vi "Ex_Inst_Read LabVIEW Measurement File.vi"(8 "error in (no error)":errorcluster, 9 "Filename":path, 10 "Enable":bool=TRUE, 11 "Reset":bool) -> (0 "error out":errorcluster, 2 "Filename Out":path, 3 "Signals":dynamicdata(graph), 4 "EOF?":bool, 5 "Comment":string, 7 "Description":string)   [LabVIEW 2017]
doc: "Reads data from a text-based measurement file (.lvm) or binary measurement file (.tdm or .tdms)."
uses:
  <vilib>/express/express shared/ExFile.llb/ex_FileFormats.ctl
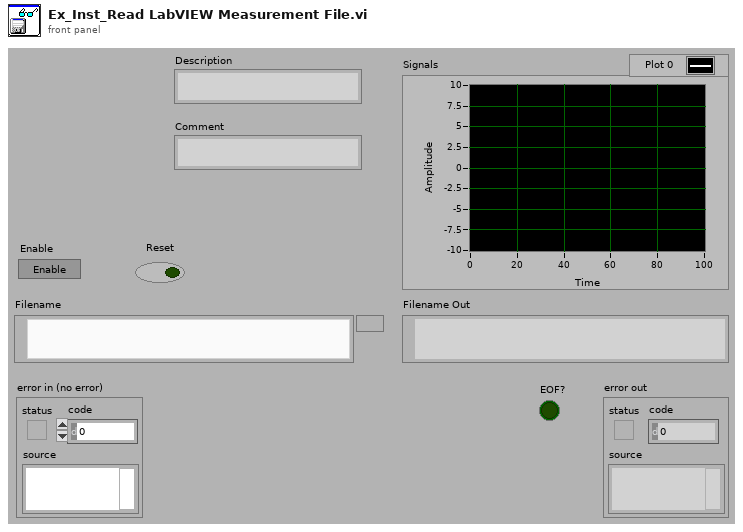
[diagram p1: front panel]
types:
  T1 = typedef "ex_FileFormats.ctl" = enum32{"lvm", "tdm", "tdms", "xlsx"}
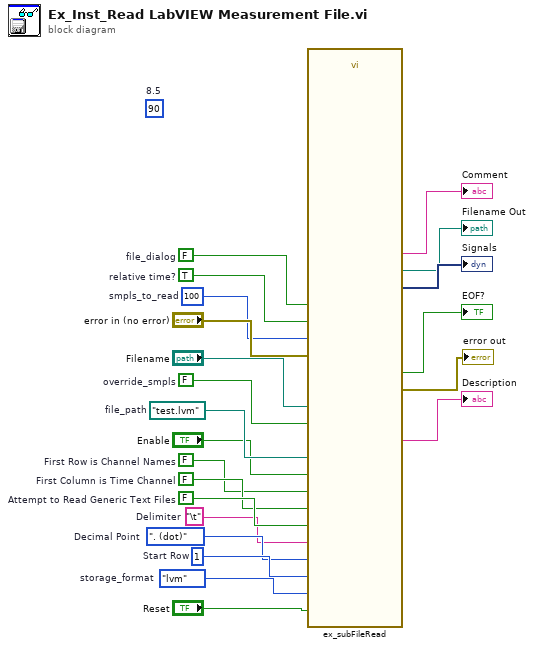
[diagram p0: block diagram]
diagram:
  (unwired) 90  # 8.5
  w4 = "\t"  # Delimiter
  w2 = ex_FileFormats."lvm"  # storage_format
  w5 = enum32{". (dot)", ", (comma)"}.". (dot)"  # Decimal Point
  w9 = 1  # Start Row
  w8 = FALSE  # Attempt to Read Generic Text Files
  w7 = FALSE  # First Column is Time Channel
  w6 = FALSE  # First Row is Channel Names
  w12 = path "test.lvm"  # file_path
  w14 = TRUE  # relative time?
  w18 = FALSE  # override_smpls
  w19 = 100  # smpls_to_read
  w20 = FALSE  # file_dialog
  n1 = call <vilib>:"ex_subFileRead.vi"("file path in"="Filename", "First Column is Time Channel"=w7, "file dialog?"=w20, "relative time?"=w14, "Attempt to Read Generic Text Files"=w8, "samples to read"=w19, "error in (no error)"="error in (no error)", "delimiter"=w4, "First Row is Channel Names"=w6, "Decimal point"=w5, "static path in"=w12, "override samples"=w18, "Enable"="Enable", "Start Row"=w9, "storage_format"=w2, "Reset"="Reset") -> ("Description"=→"Description":string, "Comment"=→"Comment":string, "EOF?"=→"EOF?":bool, "file path out"=→"Filename Out":path, "Signals"=→"Signals":dynamicdata, "error out"=→"error out":errorcluster)  [unwired: 2 in, 4 out]
